vi "Do Core.vi"(8 "error in (no error)":errorcluster, 9 "Actor in":refnum<class "Actor.lvclass">, 11 "Reply Message":refnum<class "Get SyncData Msg.lvclass">) -> (0 "error out":errorcluster, 1 "Actor out":refnum<class "Actor.lvclass">, 2 "Reply":variant)   [LabVIEW 2017, in "Filled Text Fields Actor.lvlib" / "Get SyncData Msg.lvclass"]
doc: "(<B>Filename</B>: Actor Framework.lvlib:Reply Msg.lvclass:Do Core.vi)\n\nDefines what an actor does when it receives <B>Reply Message</B>. This method also defines the <B>Reply</B> that is returned to the actor that sent <B>Reply Message</B>.\n\nBy default, this method does nothing, and <B>Reply</B> is the ancestor Message class. A child class must override this method to define behavior and specify a child of the Message class to return in the <B>Reply</B> output."
uses:
  Get SyncData Msg.lvclass
  <vilib>/ActorFramework/Actor/Actor.lvclass
  Filled Text Fields Actor/Filled Text Fields Actor.lvclass
  C:/Program Files (x86)/National Instruments/LabVIEW 2017/vi.lib/ActorFramework/Actor/Actor.lvclass
  Data/Data.lvclass
  Theme/Theme/Theme.lvclass
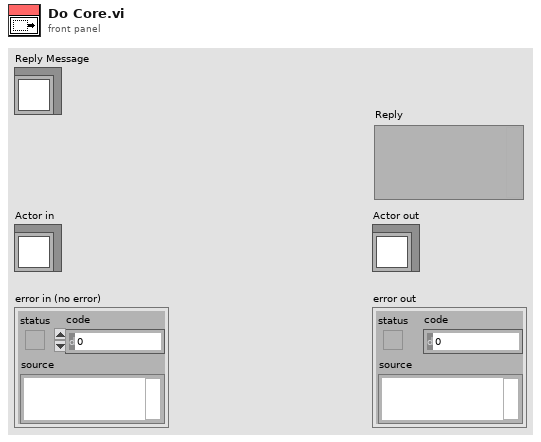
[diagram p1: front panel]
types:
  T1 = cluster{"Data":refnum<class "Data.lvclass">, "Theme":refnum<class "Theme.lvclass">}
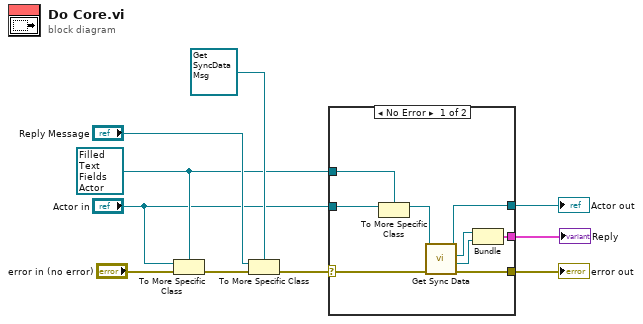
[diagram p0: block diagram]
diagram:
  w6 = refnum<class "Filled Text Fields Actor.lvclass"> refnum ("Filled Text Fields Actor.lvlib:Filled Text Fields Actor.lvclass")
  n1 = To More Specific Class(target class=w6, reference="Actor in", error in="error in (no error)") -> (error out=w10:errorcluster)  [unwired: 1 out]
  n2 = To More Specific Class(target class=refnum<class "Get SyncData Msg.lvclass"> refnum ("Filled Text Fields Actor.lvlib:Get SyncData Msg.lvclass"), reference="Reply Message", error in=w10) -> (error out=w7:errorcluster)  [unwired: 1 out]
  n3 = case shown="No Error" w7 {
    selector: w7 -> [w16 w20]
    tunnel: w6 -> [w18 _]
    tunnel: "Actor in" -> [w19 w21]
    tunnel: [w15 w21] -> w3
    tunnel: [w14 w20] -> w4
    tunnel: [w11 _] -> w2
    frame No Error {
      n4 = To More Specific Class(target class=w18, reference=w19) -> (specific class reference=w17:refnum<class "Filled Text Fields Actor.lvclass">)  [unwired: 1 in, 1 out]
      n5 = call "Get Sync Data.vi"("error in (no error)"=w16, "Filled Text Fields Actor in"=w17) -> ("error out"=w14:errorcluster, "Theme"=w12:refnum<class "Theme.lvclass">, "Data"=w13:refnum<class "Data.lvclass">, "Filled Text Fields Actor out"=w15:refnum<class "Filled Text Fields Actor.lvclass">)  [unwired: 6 in]
      n6 = Bundle("Data"=w13, "Theme"=w12) -> (w11:T1)  [unwired: 1 in]
    }
    frame Error {
    }
  }
  "error out" <- w4
  "Actor out" <- w3
  "Reply" <- w2
